vi "TxGen_Export Engine Configuration to File.vi"(11 "BIN file path":path=path "C:/Users/Administrator/Desktop/git/niveristand-aim-arinc664-custom-device/Docs/User Guide/Assets/standard_frames_udp.bin") -> (0 "error out":errorcluster)   [LabVIEW 2020]
uses:
  Frame Configuration/controls/frame_file_entry.ctl
  Frame Configuration/controls/frame_record_type.ctl
  <instrlib>/AIM GmbH/_AIM 664/_controls/queue_header_generic.ctl
  Frame Configuration/controls/Payload Record Type.ctl
  Frame Configuration/controls/Type of Payload.ctl
  Import/AIM ARINC 664 Import.lvlib
  <instrlib>/AIM GmbH/_AIM 664/AIM664LV.lvlib
panel:
  out "valids":bool[](array[boolean])
  out "Engine Configuration path out":path
  out "Engine Configuration":T1[](array[typedef])=[{"key"="Frame1", "value"={"HeaderInfo"={"InterFrameGap"=0, "PacketGroupWaitTime"=10000, "PayloadBufferMode"=0, "PayloadGenerationMode"=0, "PreambleCount"=7, "Skew"=0, "NetSelect"=3, "FrameStartMode"=1, "PhysErrorInjection"=0, "SequenceNumberInit"=65535, "SequenceNumberOffset"=65535}, "Data"=[3, 0, 0, 0, 0, 60, 2, 0, 0, 1, 33, 32, 8, 0, 69, 0, 0, 156, 0, 0, 64, 0, 1, 17, 109, 51, 10, 1, 33, 1, 224, 224, 0, 60, 0, 1, 0, 1, 0, 136, 0, 0, 183, 122, 184, 199, 167, 222, 211, 1, 45, 188, 73, 85, 5, 199, 94, 116, 211, 171, 200, 92, 39, 150, 8, 249, 210, 198, 153, 162, 103, 115, 132, 211, 215, 57, 202, 69, 106, 8, 164, 108, 196, 27, 184, 55, 219, 184, 178, 109, 147, 168, 6, 254, 10, 27, 224, 48, 172, 252, 77, 228, 65, 126, 58, 94, 41, 3, 123, 104, 241, 168, 152, 229, 217, 112, 58, 20, 194, 104, 206, 168, 100, 173, 1, 106, 54, 18, 159, 233, 167, 64, 228, 122, 132, 6, 255, 16, 150, 223, 230, 19, 165, 232, 41, 249, 88, 97, 37, 103, 92, 3, 46, 6, 10, 61, 53, 140, 59, 159, 69, 25, 50, 28, 64, 142, 126, 145, 35, 81, 0, 0, 0, 0, 0]}}] {"value"."Data" format="%.0x"; "value"."HeaderInfo"."NetSelect" items=["FDX_TX_FRAME_DLY_A"=0, "FDX_TX_FRAME_DLY_B"=1, "FDX_TX_FRAME_BOTH "=3, "FDX_TX_FRAME_ONLY_A"=4, "FDX_TX_FRAME_ONLY_B "=5]; "value"."HeaderInfo"."FrameStartMode" items=["FDX_TX_FRAME_START_IFG", "FDX_TX_FRAME_START_PGWT", "FDX_TX_FRAME_START_TRG"]; "value"."HeaderInfo"."PhysErrorInjection" items=["FDX_TX_FRAME_ERR_OFF"=0, "FDX_TX_FRAME_ERR_CRC"=1, "FDX_TX_FRAME_ERR_ALI"=2, "FDX_TX_FRAME_ERR_PRE"=4, "FDX_TX_FRAME_ERR_PHY"=8]; "value"."HeaderInfo"."SequenceNumberInit" items=["FDX_TX_FRAME_SEQ_INIT_AUTO"=65535]; "value"."HeaderInfo"."SequenceNumberOffset" items=["FDX_TX_FRAME_SEQ_OFFS_AUTO "=65535]; "value"."HeaderInfo"."PayloadGenerationMode" items=["FDX_TX_FRAME_PGM_USER"=0, "FDX_TX_FRAME_PGM_IP_PART"=1, "FDX_TX_FRAME_PGM_IP_FULL"=2, "FDX_TX_FRAME_PGM_IP_PART_TT"=10, "FDX_TX_FRAME_PGM_IP_FULL_TT"=20]; "value"."HeaderInfo"."PayloadBufferMode" items=["FDX_TX_FRAME_PBM_STD", "FDX_TX_FRAME_PBM_MAC", "FDX_TX_FRAME_PBM_UDP"]}
  in  "port index":i32
  in  "XML file path":path=path "C:/Users/Administrator/Desktop/git/niveristand-aim-arinc664-custom-device/Docs/User Guide/Assets/Loopback_TxGen_RxMonitor.xml"
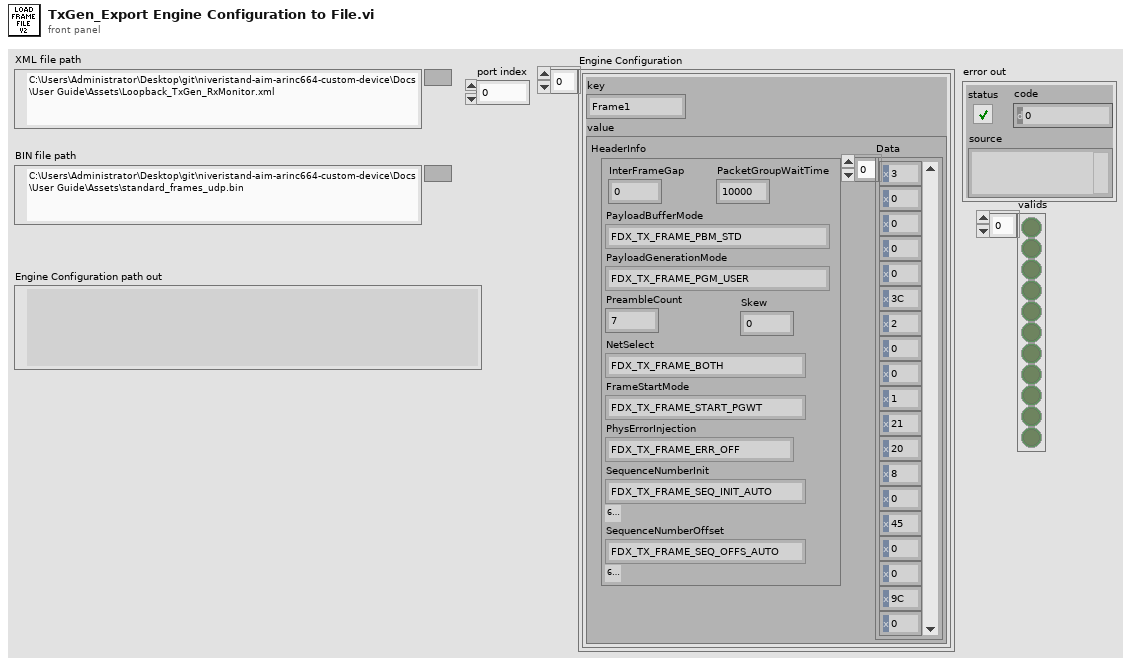
[diagram p1: front panel]
types:
  T1 = typedef "frame_file_entry.ctl" = cluster{"key":string, "value":T2}
  T2 = typedef "frame_record_type.ctl" = cluster{"HeaderInfo":T3, "Data":u8[]}
  T3 = typedef "AIM664LV.lvlib/queue_header_generic.ctl" = cluster{"InterFrameGap":u32, "PacketGroupWaitTime":u32, "PayloadBufferMode":u8, "PayloadGenerationMode":u8, "PreambleCount":u8, "Skew":u32, "NetSelect":u8, "FrameStartMode":u8, "PhysErrorInjection":u32, "SequenceNumberInit":u16, "SequenceNumberOffset":u16}
  T4 = typedef "Payload Record Type.ctl" = cluster{"Data":u8[], "Type of Frame":T5}
  T5 = typedef "Type of Payload.ctl" = u16
  T6 = typedef "AIM ARINC 664 Import.lvlib/Board Top Level Configuration.ctl" = cluster{"boardSetup":T7, "portConfiguration":T8[]}
  T7 = typedef "AIM ARINC 664 Import.lvlib/board_setup.ctl" = cluster{"boardId":u32, "portSpeed":u32, "portConfig":u32}
  T8 = typedef "AIM ARINC 664 Import.lvlib/port_configuration.ctl" = cluster{"portSetup":T9, "Tx_Generic":T10[], "Rx_Monitor":cluster{"DefaultCronoMode":u32, "GlbMonBufferSizeIn":u32, "CaptureMode":u32, "MaxFileSizeMB":u32, "Strobe":u32, "TriggerPosition":u32}[], "Tx_UDP":cluster{"tx_udp_setup":cluster{"VlId":i32, "Bag":i32, "NetSelect":u32, "domainID":u8, "sideID":u8, "locationID":u8, "interfaceID":u8, "NumOfSubVl":u16, "Skew":u32, "MaxFrameLength":u32, "FrameBufferSize":u32}, "commPorts":T18[], "sapPorts":T19[]}[], "Rx_UDP":cluster{"Tx_UDP":T20, "commPorts":T21[], "sapPorts":T22[]}[]}
  T9 = typedef "AIM ARINC 664 Import.lvlib/port_setup.ctl" = cluster{"port Id":u32, "redundant":bool}
  T10 = typedef "AIM ARINC 664 Import.lvlib/session_tx_generic.ctl" = cluster{"tx_generic_setup":T11, "Frame Headers":T12[]}
  T11 = typedef "AIM ARINC 664 Import.lvlib/tx_generic_setup.ctl" = cluster{"QueueSizeIn":u32, "Count":i32, "StartMode":i32}
  T12 = typedef "AIM ARINC 664 Import.lvlib/frame_tx_generic.ctl" = cluster{"FrameID":string, "PayloadID":string, "Frame header":cluster{"FrameStartMode":i32, "InterFrameGap":i32, "PacketGroupWaitTime":i32, "NetSelect":u32, "PayloadBufferMode":i32, "PayloadGenerationMode":i32, "PhysErrorInjection":i32, "PreambleCount":i32, "SequenceNumberInit":T13, "SequenceNumberOffset":T14, "Skew":i32}, "Parameters":T15[]}
  T13 = typedef "AIM ARINC 664 Import.lvlib/frame_tx_generic_seqNumberInit.ctl" = i32
  T14 = typedef "AIM ARINC 664 Import.lvlib/frame_tx_generic_seqNumberOffset.ctl" = i32
  T15 = typedef "AIM ARINC 664 Import.lvlib/frame_parameter.ctl" = cluster{"name":string, "default value":dbl, "unit":string, "Parameter":T16}
  T16 = typedef "AIM ARINC 664 Import.lvlib/frame_parameter_definition.ctl" = cluster{"start index":i32, "size":i32, "encoding":T17, "signed":bool, "scale multiplier":dbl, "scale offset":dbl}
  T17 = typedef "Encoding (Arinc664).ctl" = u16
  T18 = typedef "AIM ARINC 664 Import.lvlib/port_tx_udp_comm.ctl" = cluster{"PayloadID":string, "partitionID":u8, "UdpSrcPort":u16, "UdpDstPort":u16, "PortType":enum16{"FDX_UDP_SAMPLING", "FDX_UDP_QUEUING"}, "SubVIId":u32, "UdpNumBufMessages":u32, "UdpMaxMessageSize":u32, "UdpSamplingRate":u32, "Parameters":T15[]}
  T19 = typedef "AIM ARINC 664 Import.lvlib/port_tx_udp_sap.ctl" = cluster{"PayloadID":string, "SubVlId":u8, "UdpSrcPort":u16, "UdpNumBufMessages":u32, "UdpMaxMessageSize":u32, "partitionID":u8, "domainID":u8, "sideID":u8, "locationID":u8, "interfaceID":u8, "Parameters":T15[]}
  T20 = typedef "AIM ARINC 664 Import.lvlib/rx_udp_setup.ctl" = cluster{"VerificationMode":u32, "Bag":u32, "Jitter":u32, "MaxFrameLength":u32, "MaxSkew":u32, "VLBufSize":u32, "FilterMode":u32, "FilterPosition":u32, "Padding":u32, "FilterMask":u32, "FilterData":u32, "MinFrameLength":u32, "VlId":u16, "VLRange":u32}
  T21 = typedef "AIM ARINC 664 Import.lvlib/port_rx_udp_comm.ctl" = cluster{"PayloadID":string, "domainID":u8, "sideID":u8, "locationID":u8, "partitionID":u8, "UdpSrcPort":u16, "UdpDstPort":u16, "PortType":enum16{"FDX_UDP_SAMPLING", "FDX_UDP_QUEUING"}, "SubVIId":u32, "UdpNumBufMessages":u32, "UdpMaxMessageSize":u32, "UdpSamplingRate":u32, "Parameters":T15[]}
  T22 = typedef "AIM ARINC 664 Import.lvlib/port_rx_udp_sap.ctl" = cluster{"PayloadID":string, "UdpDstPort":u16, "UdpNumBufMessages":u32, "UdpMaxMessageSize":u32, "Parameters":T15[]}
  T23 = cluster{"FrameStartMode":i32, "InterFrameGap":i32, "PacketGroupWaitTime":i32, "NetSelect":u32, "PayloadBufferMode":i32, "PayloadGenerationMode":i32, "PhysErrorInjection":i32, "PreambleCount":i32, "SequenceNumberInit":T13, "SequenceNumberOffset":T14, "Skew":i32}
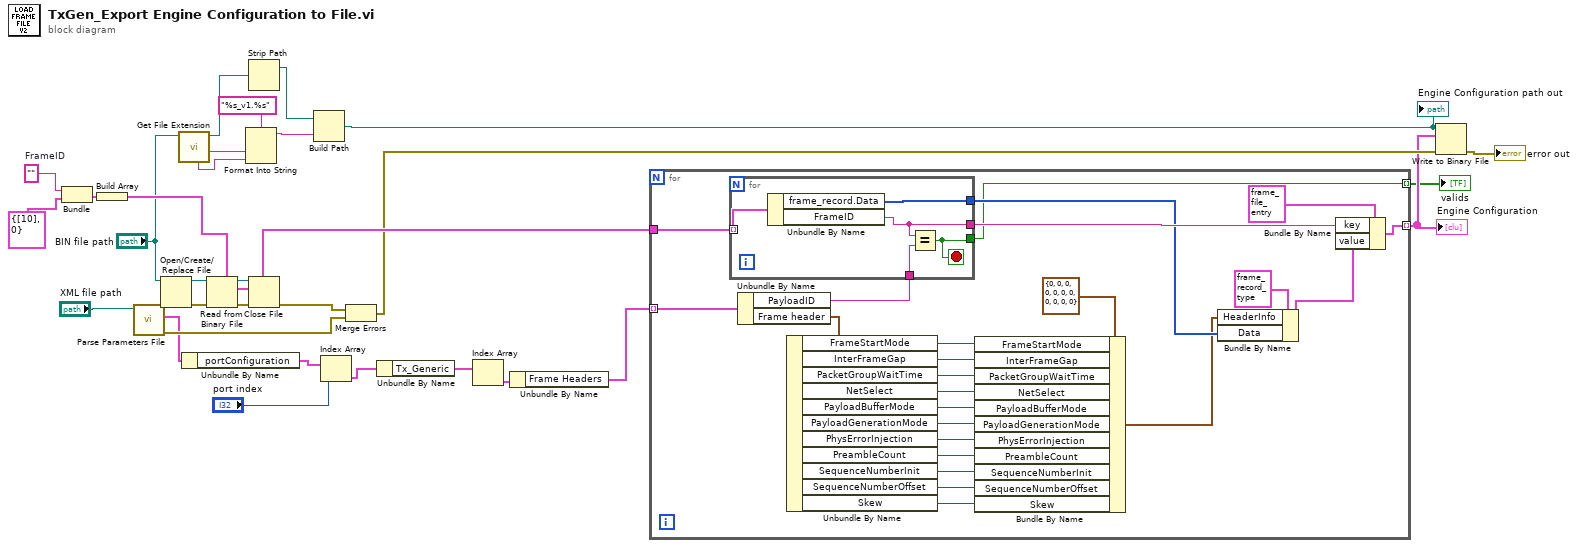
[diagram p0: block diagram]
diagram:
  w25 = ""  # FrameID
  n1 = Bundle("FrameID"=w25, "frame_record"=T4 {"Data"=[10], "Type of Frame"=0}) -> (w24:cluster{"FrameID":string, "frame_record":T4})  [unwired: 1 in]
  n2 = Build Array(w24) -> (w23:cluster{"FrameID":string, "frame_record":T4}[])
  n3 = call "Parse Parameters File.vi"("path to XML document"="XML file path") -> ("error out"=w21:errorcluster, "board configuration out"=w20:T6)  [unwired: 8 in, 1 out]
  n4 = Open/Create/Replace File(file path (use dialog)="BIN file path") -> (refnum out=w29:refnum<file>, error out=w28:errorcluster)  [unwired: 5 in, 1 out]
  n5 = call <vilib>:"Get File Extension.vi"("file"="BIN file path") -> ("filename without extension"=w13:string, "dup file"=w11:path, "unmodified file extension"=w10:string)  [unwired: 6 in, 2 out]
  n6 = Unbundle By Name(w20) -> ("portConfiguration"=w19:T8[])
  n7 = Read from Binary File(5:w23, 8:w28, 11:w29) -> (0:w30:errorcluster, 2:w6:cluster{"FrameID":string, "frame_record":T4}[], 3:w31:refnum<file>)  [unwired: 3 in, 1 out]
  n8 = Format Into String(format string="%s_v1.%s", w13, w10) -> (resulting string=w8:string)  [unwired: 2 in, 1 out]
  n9 = Strip Path(path=w11) -> (stripped path=w9:path)  [unwired: 1 out]
  n10 = Close File(refnum=w31, error in=w30) -> (error out=w27:errorcluster)  [unwired: 1 out]
  n11 = Build Path(base path=w9, name or relative path=w8) -> (appended path=w7:path)
  "Engine Configuration path out" <- w7
  n12 = Index Array(array=w19, index="port index") -> (element=w18:T8)
  n13 = Merge Errors(w27, w21) -> (w4:errorcluster)
  n14 = Unbundle By Name(w18) -> ("Tx_Generic"=w16:T10[])
  n15 = Index Array(array=w16) -> (element=w15:T10)  [unwired: 1 in]
  n16 = Unbundle By Name(w15) -> ("Frame Headers"=w5:T12[])
  n17 = for {
    tunnel: w6 -> [w53]
    tunnel: w5 -> [w52] mode=indexing
    tunnel: [w54] -> w3 mode=indexing
    tunnel: [w32] -> w1 mode=indexing
    n18 = Unbundle By Name(w52) -> ("PayloadID"=w33:string, "Frame header"=w47:T23)
    n19 = for {
      tunnel: w53 -> [w60] mode=indexing
      tunnel: [w57] -> w49
      tunnel: [w59] -> w48
      tunnel: w33 -> [w58]
      tunnel: [w56] -> w32
      stop <- w56 stop-if-true
      n20 = Unbundle By Name(w60) -> ("frame_record.Data"=w59:u8[], "FrameID"=w57:string)
      n21 = Equal?(x=w57, y=w58) -> (x = y?=w56:bool)
    }
    n22 = Unbundle By Name(w47) -> ("FrameStartMode"=w44:i32, "InterFrameGap"=w43:i32, "PacketGroupWaitTime"=w42:i32, "NetSelect"=w41:u32, "PayloadBufferMode"=w40:i32, "PayloadGenerationMode"=w39:i32, "PhysErrorInjection"=w38:i32, "PreambleCount"=w37:i32, "SequenceNumberInit"=w36:T13, "SequenceNumberOffset"=w35:T14, "Skew"=w34:i32)
    n23 = Bundle By Name(cluster=T3 {"InterFrameGap"=0, "PacketGroupWaitTime"=0, "PayloadBufferMode"=0, "PayloadGenerationMode"=0, "PreambleCount"=0, "Skew"=0, "NetSelect"=0, "FrameStartMode"=0, "PhysErrorInjection"=0, "SequenceNumberInit"=0, "SequenceNumberOffset"=0} ("HeaderInfo"), "FrameStartMode"=w44, "InterFrameGap"=w43, "PacketGroupWaitTime"=w42, "NetSelect"=w41, "PayloadBufferMode"=w40, "PayloadGenerationMode"=w39, "PhysErrorInjection"=w38, "PreambleCount"=w37, "SequenceNumberInit"=w36, "SequenceNumberOffset"=w35, "Skew"=w34) -> (w45:T3)
    n24 = Bundle By Name(cluster=T2 {"HeaderInfo"={"InterFrameGap"=0, "PacketGroupWaitTime"=10000, "PayloadBufferMode"=0, "PayloadGenerationMode"=0, "PreambleCount"=7, "Skew"=0, "NetSelect"=4, "FrameStartMode"=1, "PhysErrorInjection"=0, "SequenceNumberInit"=65535, "SequenceNumberOffset"=65535}, "Data"=[10]} ("value"), "HeaderInfo"=w45, "Data"=w48) -> (w50:T2)
    n25 = Bundle By Name(cluster=T1 {"key"="", "value"={"HeaderInfo"={"InterFrameGap"=0, "PacketGroupWaitTime"=0, "PayloadBufferMode"=0, "PayloadGenerationMode"=0, "PreambleCount"=0, "Skew"=0, "NetSelect"=0, "FrameStartMode"=0, "PhysErrorInjection"=0, "SequenceNumberInit"=0, "SequenceNumberOffset"=0}, "Data"=[]}} ("v1 Data 2"), "key"=w49, "value"=w50) -> (w54:T1)
  }
  "Engine Configuration" <- w3
  "valids" <- w1
  n26 = Write to Binary File(file (use dialog)=w7, data=w3, error in=w4) -> (error out=→"error out":errorcluster)  [unwired: 3 in, 2 out]
